vi "Write ID.vi"(8 "error in (no error)":errorcluster, 10 "ID":T1, 11 "ID in":refnum<class "ID.lvclass">) -> (0 "error out":errorcluster, 3 "ID out":refnum<class "ID.lvclass">)   [LabVIEW 2023, in "ID.lvclass"]
uses:
  ID.lvclass
  Controller/Ctrl_ID.ctl
  ID.lvclass/ID.ctl
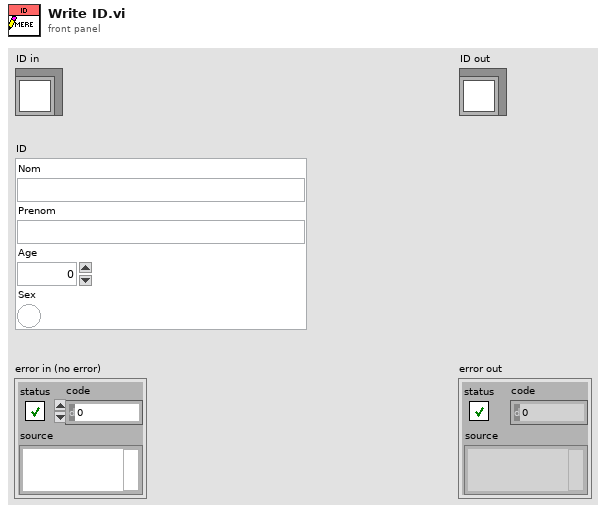
[diagram p1: front panel]
types:
  T1 = typedef "Ctrl_ID.ctl" = cluster{"Nom":string, "Prenom":string, "Age":u8, "Sex":bool}
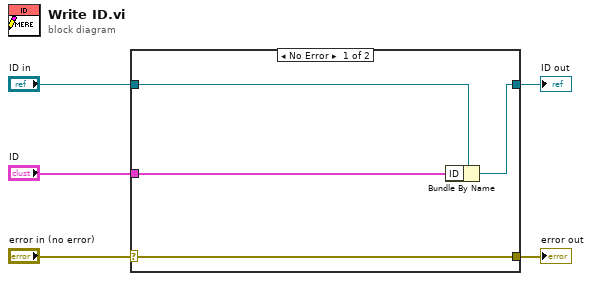
[diagram p0: block diagram]
diagram:
  n1 = case shown="No Error" "error in (no error)" {
    selector: "error in (no error)" -> [w9 w10]
    tunnel: [w9 w10] -> w4
    tunnel: [w7 w11] -> w2
    tunnel: "ID in" -> [w8 w11]
    tunnel: "ID" -> [w6 _]
    frame No Error {
      n2 = Bundle By Name(cluster=w8, "ID"=w6) -> (w7:refnum<class "ID.lvclass">)
    }
    frame Error {
    }
  }
  "error out" <- w4
  "ID out" <- w2
